vi "APS set vao table.vi"(5 "MappingDataArray":i32, 6 "TotalPoints":i32, 7 "VelInterval":i32, 8 "error in (no error)":errorcluster caption="错误输入（无错误）", 9 "MinVelocity":i32, 10 "Table_No":i32, 11 "Board_ID":i32) -> (0 "error out":errorcluster caption="错误输出", 2 "function return":i32, 3 "MappingDataArray out":i32)   [LabVIEW 2011, in "APS168.lvlib"]
doc: "I32 FNTYPE APS_set_vao_table( I32 Board_ID, I32 Table_No, I32 MinVelocity, I32 VelInterval, I32 TotalPoints, I32 *MappingDataArray );"
uses:
  APS168.lvlib
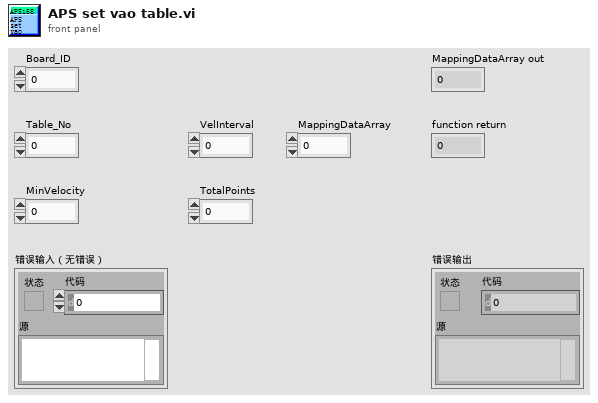
[diagram p1: front panel]
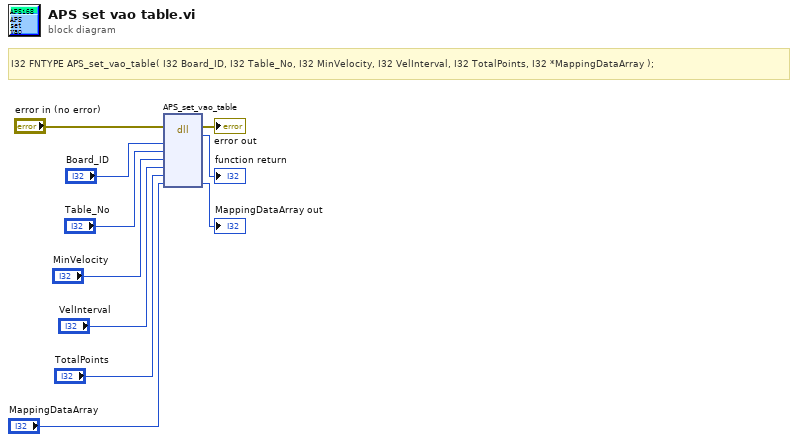
[diagram p0: block diagram]
diagram:
  # "I32 FNTYPE APS_set_vao_table( I32 Board_ID, I32 Table_No, I32 MinVelocity, I32 VelInterval, I32 TotalPoints, I32 *MappingDataArray );"
  n1 = dll-call lib="PTH1Labs E软件ADLINK 204CAPS_1_7_1_LIB line 连续运动204APS168.*" fn="APS_set_vao_table"(error in="error in (no error)", "Board_ID"="Board_ID", "Table_No"="Table_No", "MinVelocity"="MinVelocity", "VelInterval"="VelInterval", "TotalPoints"="TotalPoints", "MappingDataArray"="MappingDataArray") -> (error out=→"error out":errorcluster, →"function return":i32, "MappingDataArray"=→"MappingDataArray out":i32)  [unwired: 7 in, 1 out]
